vi "CI_AmountOfDiskUsed.vi"(0 "Display State In":T1={"StandardColor"=6881066, "WarningColor"=16766208, "CriticalColor"=15671808, "Standard<>Warning Range"=75, "Warning<>Critical Range"=95}, 5 "VolumeToMonitor":path, 9 "Container State":T2, 11 "error in (no error)":errorcluster) -> (4 "Display State Out":T1={"StandardColor"=6881066, "WarningColor"=16766208, "CriticalColor"=15671808, "Standard<>Warning Range"=75, "Warning<>Critical Range"=95}, 15 "error out":errorcluster)   [LabVIEW 2010, in "CapacityIndicator.xctl"]
doc: "Get percent of disk used."
uses:
  CapacityIndicator.xctl
  <vilib>/_xctls/Container State.ctl
  CI_State.ctl
  <vilib>/_xctls/XControlSupport.lvlib
panel:
  # "Add Controls & Indicators that form the parameters of the method here. Hook them to the connector pane. Do not delete the controls & indicators that are already hooked to the connector pane.\n \nTo setup the parameters  for this method, right click on this item in the Project Tree & select \"Configure Method...\"."
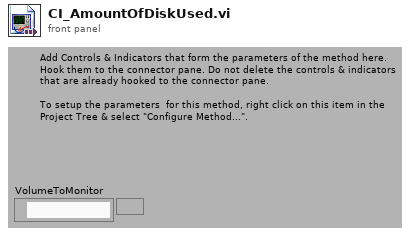
[diagram p1: front panel]
types:
  T1 = typedef "CapacityIndicator.xctl/CI_State.ctl" = cluster{"StandardColor":u32, "WarningColor":u32, "CriticalColor":u32, "Standard<>Warning Range":u8, "Warning<>Critical Range":u8}
  T2 = typedef "XControlSupport.lvlib/Container State.ctl" = cluster{"Indicator?":bool, "Run Mode?":bool, " Refnum":refnum<vi>}
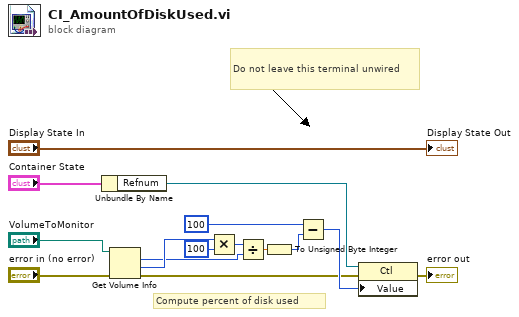
[diagram p0: block diagram]
diagram:
  # "Compute percent of disk used"
  # "Do not leave this terminal unwired"
  n1 = Unbundle By Name("Container State") -> ("Refnum"=w4:refnum<vi>)
  n2 = Get Volume Info(8:"error in (no error)", 11:"VolumeToMonitor") -> (0:w1:errorcluster, 1:w11:i64, 2:w8:i64)  [unwired: 3 out]
  n3 = Multiply(x=w11, y=i64 100) -> (x*y=w9:i64)
  n4 = Divide(x=w9, y=w8) -> (x/y=w7:dbl)
  n5 = To Unsigned Byte Integer(number=w7) -> (unsigned 8bit integer=w6:u8)
  n6 = Subtract(x=u8 100, y=w6) -> (x-y=w3:u8)
  n7 = property class="Ctl"(reference=w4, error in=w1, "Value"=w3) -> (error out=→"error out":errorcluster)  [unwired: 1 out]
  "Display State Out" <- "Display State In"
